vi "CRYReport Pic Find Frame.vi"(7 "sAction":string, 8 "nData":i32, 9 "sData":string) -> (0 "nData_Out":i32, 3 "cFrame_Out":T1)   [LabVIEW 2013]
uses:
  CRYReport Global.vi
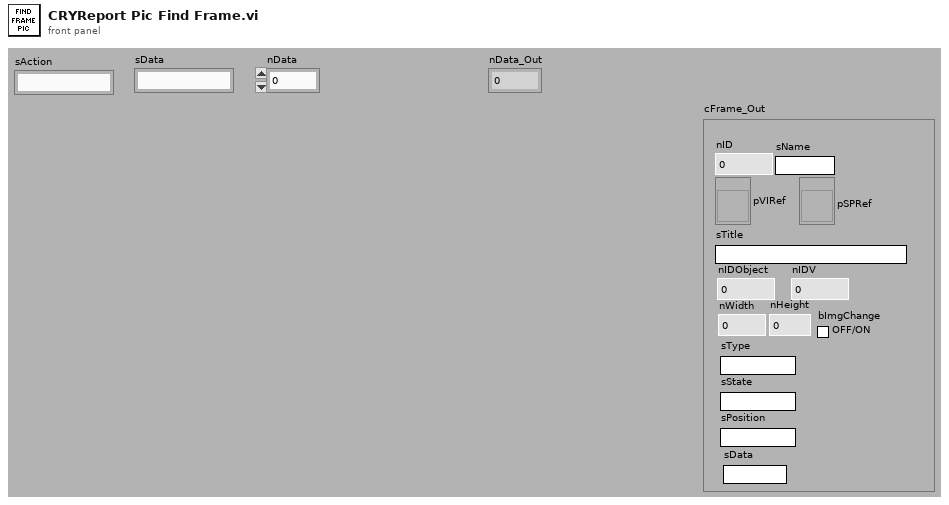
[diagram p1: front panel]
types:
  T1 = cluster{"nID":i16, "sName":string, "pVIRef":refnum<vi>, "pSPRef":refnum<vi>, "sTitle":string, "nIDObject":i16, "nIDV":i16, "nWidth":i16, "nHeight":i16, "bImgChange":bool, "sType":string, "sState":string, "sPosition":string, "sData":string}
  T2 = cluster{"nCount":i16, "cFrameList":cluster{"nID":i16, "sName":string, "pVIRef":refnum<vi>, "pSPRef":refnum<vi>, "sTitle":string, "nIDObject":i16, "nIDV":i16, "nWidth":i16, "nHeight":i16, "bImgChange":bool, "sType":string, "sState":string, "sPosition":string, "sData":string}[], "sData":string}
  T3 = cluster{"nID":i16, "sName":string, "pVIRef":refnum<vi>, "pSPRef":refnum<vi>, "sTitle":string, "nIDObject":i16, "nIDV":i16, "nWidth":i16, "nHeight":i16, "bImgChange":bool, "sType":string, "sState":string, "sPosition":string, "sData":string}[]
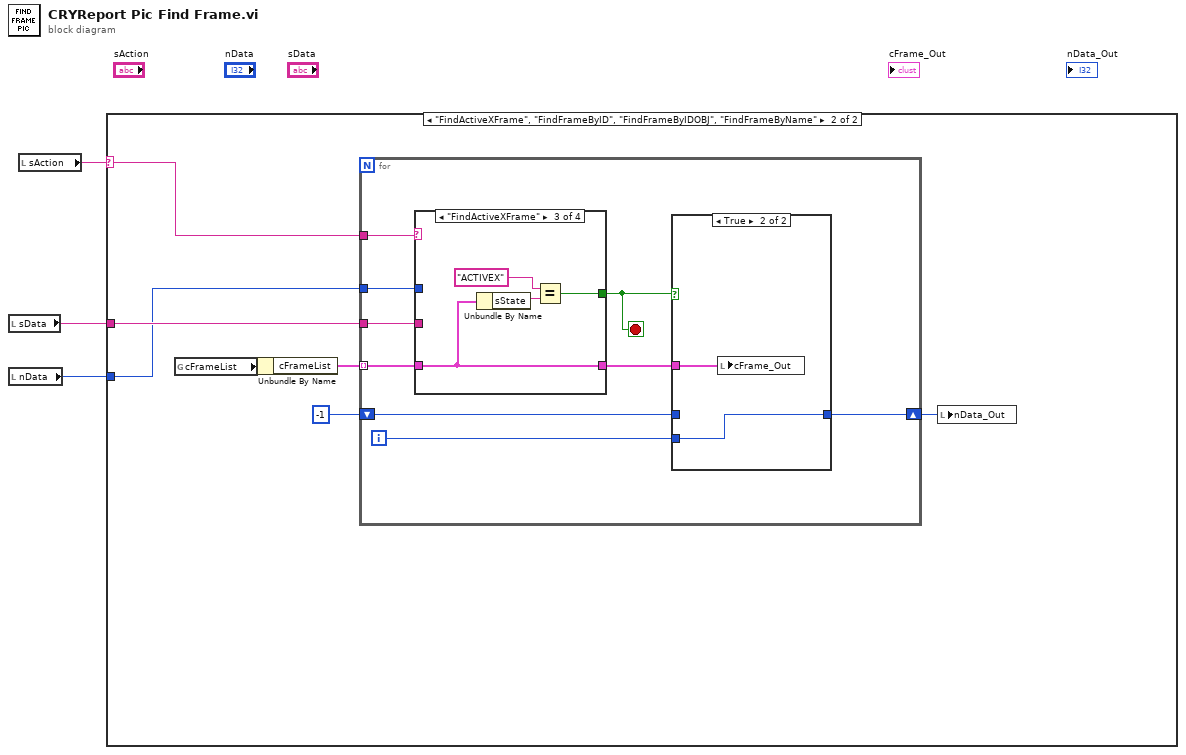
[diagram p0: block diagram]
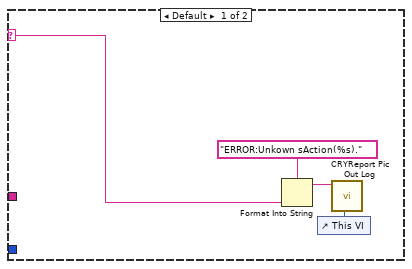
[diagram p2: hidden frame]
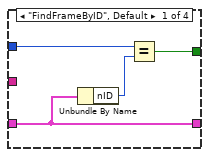
[diagram p4: hidden frame]
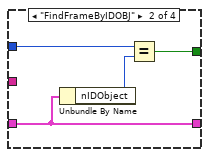
[diagram p5: hidden frame]
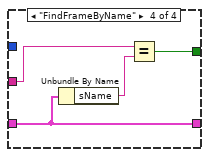
[diagram p6: hidden frame]
diagram:
  n1 = local read "sData"() -> (w2:string)
  n2 = local read "nData"() -> (w1:i32)
  n3 = local read "sAction"() -> (w3:string)
  n4 = case shown="\"FindActiveXFrame\", \"FindFrameByID\", \"FindFrameByIDOBJ\", \"FindFrameByName\"" w3 {
    selector: w3 -> [w5 w12]
    tunnel: w2 -> [_ w11]
    tunnel: w1 -> [_ w10]
    frame Default {
      n5 = Format Into String(format string="ERROR:Unkown sAction(%s).", w5) -> (resulting string=w4:string)  [unwired: 2 in, 1 out]
      n6 = control-ref of="This VI"() -> (w7:refnum<vi>)
      n7 = call "CRYReport Pic Out Log.vi"("vi reference"=w7, "sData"=w4) -> ()  [unwired: 10 in]
    }
    frame "FindActiveXFrame", "FindFrameByID", "FindFrameByIDOBJ", "FindFrameByName" {
      n8 = global read "CRYReport Global.vi" "cFrameList"() -> (w14:T2)
      n9 = Unbundle By Name(w14) -> ("cFrameList"=w13:T3)
      n10 = for {
        tunnel: w10 -> [w22]
        tunnel: w13 -> [w21] mode=indexing
        tunnel: w12 -> [w23]
        tunnel: w11 -> [w18]
        shift-right: [w15] -> w8
        shift-left: -1 -> [w17]
        i -> [w16]
        stop <- w19 stop-if-true
        n11 = case shown="\"FindActiveXFrame\"" w23 {
          tunnel: w22 -> [w29 w33 _ _]
          tunnel: w21 -> [w27 w31 w37 w40]
          tunnel: [w28 w32 w38 w41] -> w19
          tunnel: [w27 w31 w37 w40] -> w20
          tunnel: w18 -> [_ _ _ w39]
          frame "FindFrameByID", Default {
            n12 = Unbundle By Name(w27) -> ("nID"=w30:i16)
            n13 = Equal?(x=w29, y=w30) -> (x = y?=w28:bool)
          }
          frame "FindFrameByIDOBJ" {
            n14 = Unbundle By Name(w31) -> ("nIDObject"=w34:i16)
            n15 = Equal?(x=w33, y=w34) -> (x = y?=w32:bool)
          }
          frame "FindActiveXFrame" {
            n16 = Unbundle By Name(w37) -> ("sState"=w36:string)
            n17 = Equal?(x="ACTIVEX", y=w36) -> (x = y?=w38:bool)
          }
          frame "FindFrameByName" {
            n18 = Unbundle By Name(w40) -> ("sName"=w42:string)
            n19 = Equal?(x=w39, y=w42) -> (x = y?=w41:bool)
          }
        }
        n20 = case shown="True" w19 {
          tunnel: w20 -> [_ w26]
          tunnel: w17 -> [w24 _]
          tunnel: w16 -> [_ w25]
          tunnel: [w24 w25] -> w15
          frame False {
          }
          frame True {
            n21 = local write "cFrame_Out"(w26) -> ()
          }
        }
      }
      n22 = local write "nData_Out"(w8) -> ()
    }
  }
